vi "Sensor Persistence State.vi"(10 "Sensor":bool, 11 "Pump State in":bool) -> (2 "Persistent State":bool, 3 "Pump State out":bool)   [LabVIEW 2018]
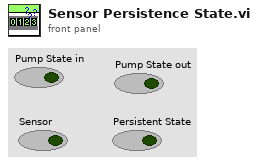
[diagram p1: front panel]
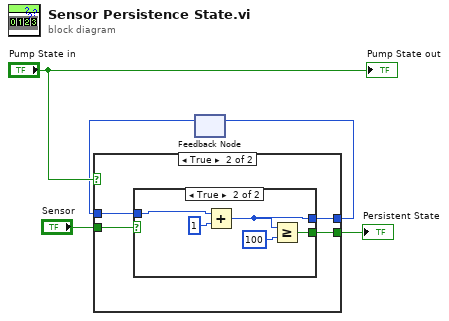
[diagram p0: block diagram]
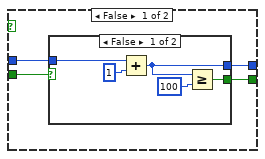
[diagram p2: hidden frame]
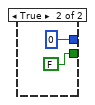
[diagram p3: hidden frame]
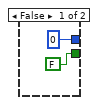
[diagram p4: hidden frame]
diagram:
  n1 = feedback #1() -> (w4:i32)  [unwired: 1 in]
  n2 = case shown="True" "Pump State in" {
    tunnel: "Sensor" -> [w8 w20]
    tunnel: w4 -> [w9 w19]
    tunnel: [w6 w18] -> w3
    tunnel: [w7 w17] -> w2
    frame False {
      n3 = case shown="False" w8 {
        tunnel: w9 -> [w14 _]
        tunnel: [w12 0] -> w6
        tunnel: [w10 FALSE] -> w7
        frame False {
          n4 = Add(x=w14, y=1) -> (x+y=w12:i32)
          n5 = Greater Or Equal?(x=w12, y=100) -> (x >= y?=w10:bool)
        }
        frame True {
        }
      }
    }
    frame True {
      n6 = case shown="True" w20 {
        tunnel: w19 -> [_ w27]
        tunnel: [0 w25] -> w18
        tunnel: [FALSE w23] -> w17
        frame False {
        }
        frame True {
          n7 = Add(x=w27, y=1) -> (x+y=w25:i32)
          n8 = Greater Or Equal?(x=w25, y=100) -> (x >= y?=w23:bool)
        }
      }
    }
  }
  "Persistent State" <- w2
  n9 = feedback-in #1(w3) -> ()
  "Pump State out" <- "Pump State in"
